vi "Testing (not part of comp).vi"() -> ()   [LabVIEW 2013]
panel:
  in  "Down":bool
  in  "Up":bool
  in  "ON/OFF":bool
  in  "Return":bool
  in  "stop":bool
  in  "4 ft":bool
  # "Pickup"
  # "LED"
  # "Shooter"
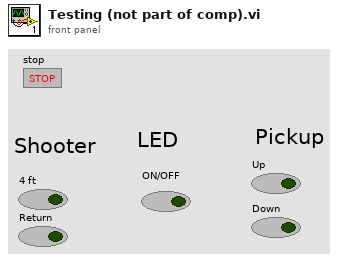
[diagram p1: front panel]
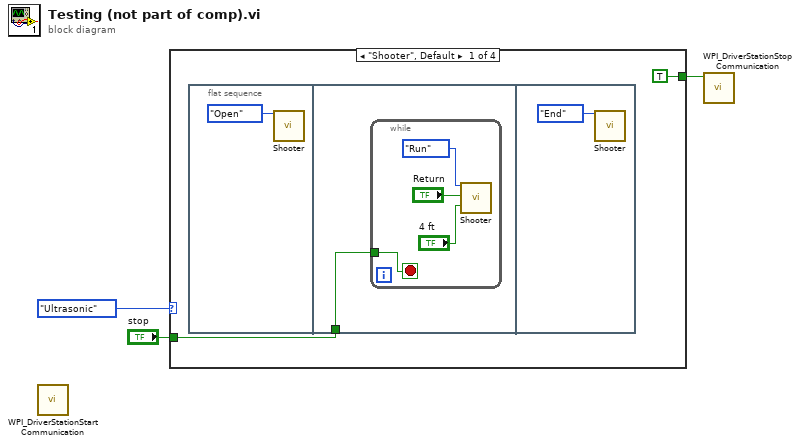
[diagram p0: block diagram]
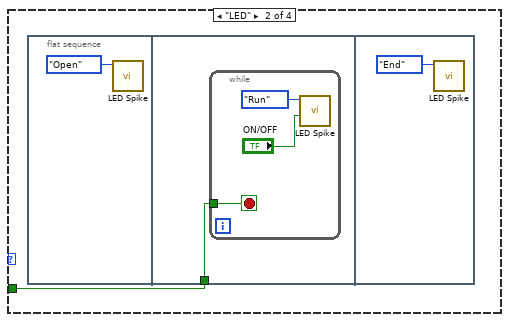
[diagram p2: hidden frame]
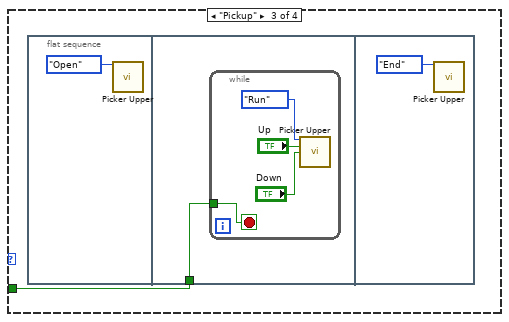
[diagram p3: hidden frame]
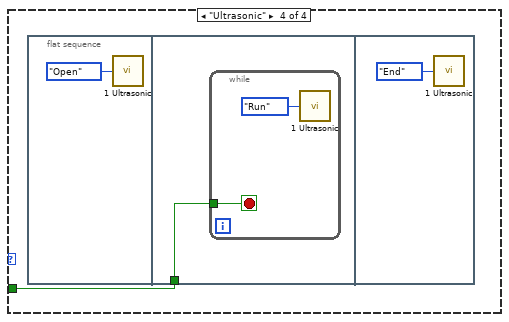
[diagram p4: hidden frame]
diagram:
  n1 = call <vilib>:"WPI_DriverStationStart Communication.vi"() -> ()  [unwired: 12 in]
  n2 = case shown="\"Shooter\", Default" enum16{"Shooter", "LED", "Ultrasonic", "Pickup"}."Ultrasonic" ("Enum") {
    tunnel: "stop" -> [w5 w13 w20 w28]
    tunnel: [TRUE _ _ _] -> w1
    frame "Shooter", Default {
      n3 = flat-sequence {
        tunnel: w5 -> [w7]
        frame #0 {
          n4 = call "Shooter.vi"("State Control"=enum16{"Open", "Run", "End"}."Open") -> ()  [unwired: 17 in, 2 out]
        }
        frame #1 {
          n5 = while {
            tunnel: w7 -> [w9]
            stop <- w9 stop-if-true
            n6 = call "Shooter.vi"("State Control"=enum16{"Open", "Run", "End"}."Run", "Return"="Return", "4 ft"="4 ft") -> ()  [unwired: 15 in, 2 out]
          }
        }
        frame #2 {
          n7 = call "Shooter.vi"("State Control"=enum16{"Open", "Run", "End"}."End") -> ()  [unwired: 17 in, 2 out]
        }
      }
    }
    frame "LED" {
      n8 = flat-sequence {
        tunnel: w13 -> [w15]
        frame #0 {
          n9 = call "LED Spike.vi"("State"=enum16{"Open", "Run", "End"}."Open" ("State Control")) -> ()  [unwired: 11 in]
        }
        frame #1 {
          n10 = while {
            tunnel: w15 -> [w18]
            stop <- w18 stop-if-true
            n11 = call "LED Spike.vi"("ON/OFF"="ON/OFF", "State"=enum16{"Open", "Run", "End"}."Run" ("State Control")) -> ()  [unwired: 10 in]
          }
        }
        frame #2 {
          n12 = call "LED Spike.vi"("State"=enum16{"Open", "Run", "End"}."End" ("State Control")) -> ()  [unwired: 11 in]
        }
      }
    }
    frame "Pickup" {
      n13 = flat-sequence {
        tunnel: w20 -> [w22]
        frame #0 {
          n14 = call "Picker Upper.vi"("State Control"=enum16{"Open", "Run", "End"}."Open") -> ()  [unwired: 13 in, 2 out]
        }
        frame #1 {
          n15 = while {
            tunnel: w22 -> [w26]
            stop <- w26 stop-if-true
            n16 = call "Picker Upper.vi"("State Control"=enum16{"Open", "Run", "End"}."Run", "Up"="Up", "Down"="Down") -> ()  [unwired: 11 in, 2 out]
          }
        }
        frame #2 {
          n17 = call "Picker Upper.vi"("State Control"=enum16{"Open", "Run", "End"}."End") -> ()  [unwired: 13 in, 2 out]
        }
      }
    }
    frame "Ultrasonic" {
      n18 = flat-sequence {
        tunnel: w28 -> [w30]
        frame #0 {
          n19 = call "1 Ultrasonic.vi"("State Control"=enum16{"Open", "Run", "End"}."Open") -> ()  [unwired: 1 out]
        }
        frame #1 {
          n20 = while {
            tunnel: w30 -> [w32]
            stop <- w32 stop-if-true
            n21 = call "1 Ultrasonic.vi"("State Control"=enum16{"Open", "Run", "End"}."Run") -> ()  [unwired: 1 out]
          }
        }
        frame #2 {
          n22 = call "1 Ultrasonic.vi"("State Control"=enum16{"Open", "Run", "End"}."End") -> ()  [unwired: 1 out]
        }
      }
    }
  }
  n23 = call <vilib>:"WPI_DriverStationStop Communication.vi"("StopCommunication"=w1) -> ()  [unwired: 10 in, 1 out]
